vi "HEWH Intellifaucet Temp Equation.vi"(8 "Error In":errorcluster, 10 "mA to F":dbl, 11 "Temp/GPM Target":dbl) -> (0 "Error Out":errorcluster, 2 "Temp (F)":dbl, 3 "Temp uA":i32)   [LabVIEW 2020]
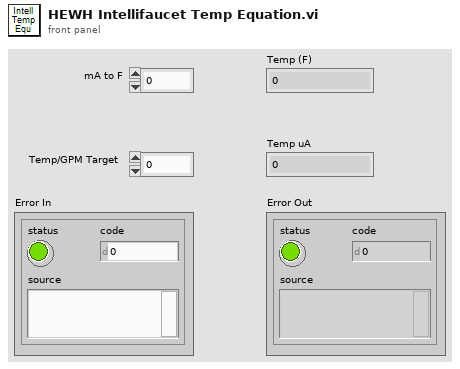
[diagram p1: front panel]
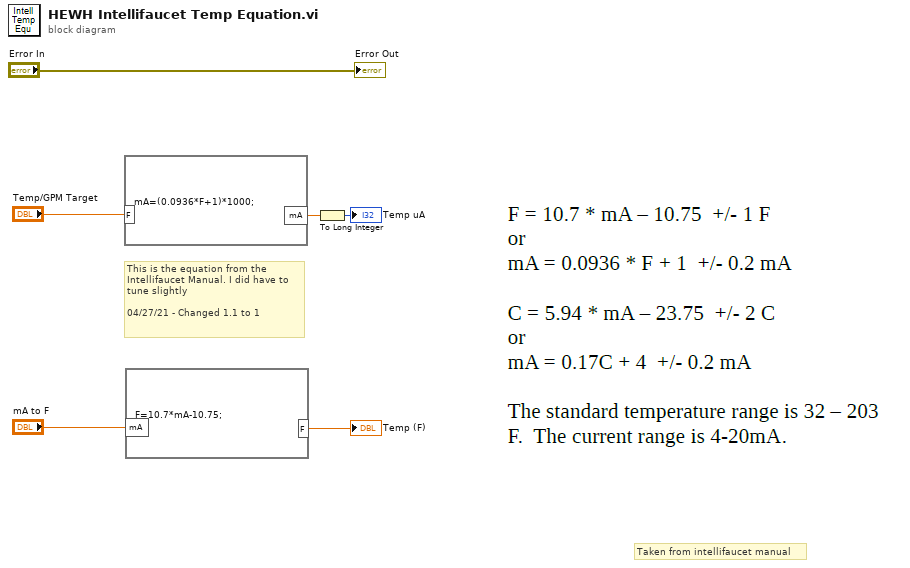
[diagram p0: block diagram]
diagram:
  # "Taken from intellifaucet manual"
  # "This is the equation from the \nIntellifaucet Manual. I did have to\ntune slightly\n\n04/27/21 - Changed 1.1 to 1"
  n1 = formula code="mA=(0.0936*F+1)*1000;"("F"="Temp/GPM Target") -> ("mA"=w5:dbl)
  n2 = formula code="F=10.7*mA-10.75;"("mA"="mA to F") -> ("F"=→"Temp (F)":dbl)
  n3 = To Long Integer(number=w5) -> (32bit integer=→"Temp uA":i32)
  "Error Out" <- "Error In"
